vi "VoltMeter.vi"(2 "NXT":T2={"Hardware"="NXT", "Flattened String"=""}, 3 "Input Port":T1 items=["Port 1", "Port 2", "Port 3", "Port 4"]) -> (1 "MilliVolts":i16, 4 "NXT dup":T2={"Hardware"="NXT", "Flattened String"=""} caption="NXT")   [LabVIEW 2010]
uses:
  <vilib>/NXT/Subs/LVHSConnector.ctl
  <vilib>/NXT/Block Support/NXT_InputPort.ctl
  <vilib>/NXT/Block Support/HWPage.SensorType.ctl
  <vilib>/NXT/Block Support/HWPage.SensorMode.ctl
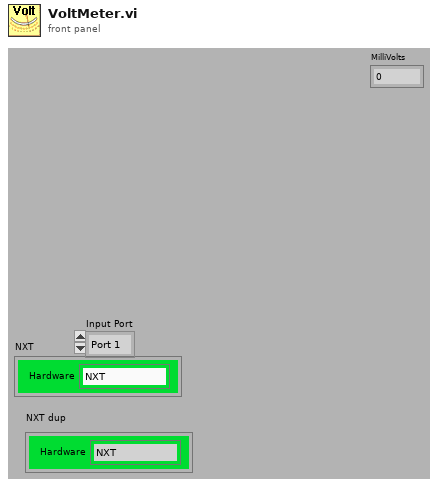
[diagram p1: front panel]
types:
  T1 = typedef "NXT_InputPort.ctl" = u8
  T2 = typedef "LVHSConnector.ctl" = cluster{"Hardware":string, "Flattened String":string}
  T3 = typedef "HWPage.SensorType.ctl" = u8
  T4 = typedef "HWPage.SensorMode.ctl" = u8
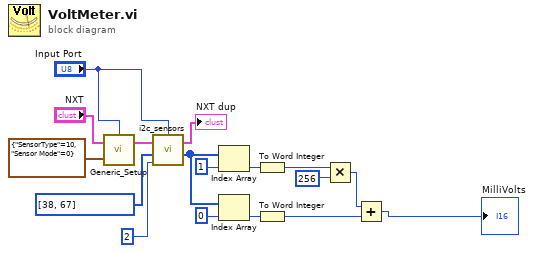
[diagram p0: block diagram]
diagram:
  n1 = call <vilib>:"Generic_Setup.vi"("Sensor Setup"=cluster{"SensorType":T3, "Sensor Mode":T4} {"SensorType"=10, "Sensor Mode"=0}, "NXT"="NXT", "Port"="Input Port") -> ("NXT"=w9:T2)  [unwired: 1 out]
  n2 = call <vilib>:"i2c_sensors.vi"("Return Length"=u8 2, "Bytes to Write"=u8[] [38, 67] ("Buffer"), "NXT"=w9, "Port"="Input Port") -> ("Bytes read"=w8:u8[], "NXT"=→"NXT dup":T2)  [unwired: 1 in, 1 out]
  n3 = Index Array(array=w8, index=1) -> (element=w6:u8)
  n4 = Index Array(array=w8, index=0) -> (element=w3:u8)
  n5 = To Word Integer(number=w6) -> (16bit integer=w2:i16)
  n6 = To Word Integer(number=w3) -> (16bit integer=w4:i16)
  n7 = Multiply(x=w2, y=256) -> (x*y=w5:i32)
  n8 = Add(x=w5, y=w4) -> (x+y=→"MilliVolts":i32)
